vi "VI_Defer FP Updata.vi"(8 "error in":errorcluster, 10 "Defer updata?":bool, 11 "Vi reference":refnum<vi>) -> (0 "错误输出":errorcluster caption="error out", 3 "Vi reference out":refnum<vi>)   [LabVIEW 2016]
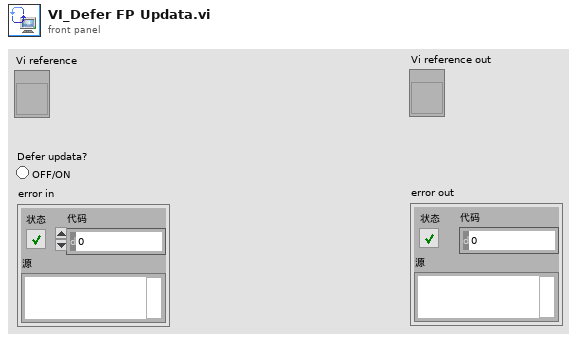
[diagram p1: front panel]
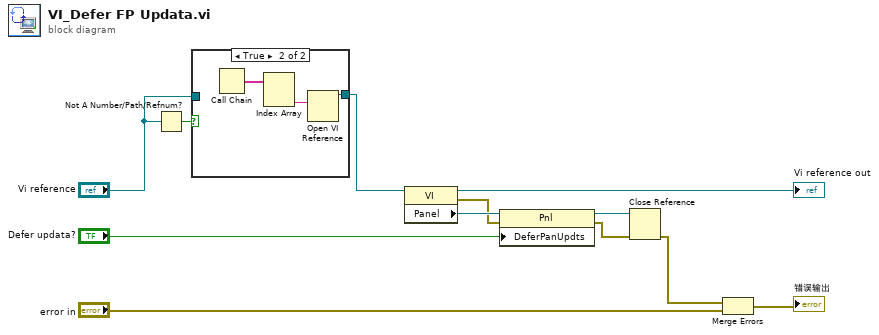
[diagram p0: block diagram]
diagram:
  n1 = Not A Number/Path/Refnum?(number/path/refnum="Vi reference") -> (NaN/Path/Refnum?=w3:bool)
  n2 = case shown="True" w3 {
    tunnel: [w13 w16] -> w1
    tunnel: "Vi reference" -> [w13 _]
    frame False {
    }
    frame True {
      n3 = Call Chain() -> (call chain=w15:string[])
      n4 = Index Array(array=w15) -> (element #2=w14:string)  [unwired: 2 in, 1 out]
      n5 = Open VI Reference(vi path=w14) -> (vi reference=w16:refnum<vi>)  [unwired: 5 in, 1 out]
    }
  }
  n6 = property class="VI"(reference=w1) -> (reference out=→"Vi reference out":refnum<vi>, error out=w11:errorcluster, "Panel"=w12:refnum<vi>)  [unwired: 1 in]
  n7 = property class="Pnl"(reference=w12, error in=w11, "DeferPanUpdts"="Defer updata?") -> (reference out=w10:refnum<vi>, error out=w9:errorcluster)
  n8 = Close Reference(reference=w10, error in (no error)=w9) -> (error out=w6:errorcluster)
  n9 = Merge Errors(w6, "error in") -> (→"错误输出":errorcluster)
